vi "Get CAN Task Events.vi"(11 "CANopen Master in":refnum<class "CANopen Master.lvclass">) -> (2 "CAN Task Events":T1, 3 "CANopen Master out":refnum<class "CANopen Master.lvclass">)   [LabVIEW 2024, in "CANopen Master.lvlib" / "CANopen Master.lvclass"]
uses:
  CANopen Master.lvclass
  CANopen Master.lvclass/CANopen Master.ctl
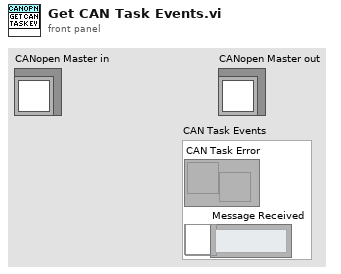
[diagram p1: front panel]
types:
  T1 = cluster{"CAN Task Error":refnum<user-event>, "Message Received":refnum<user-event>}
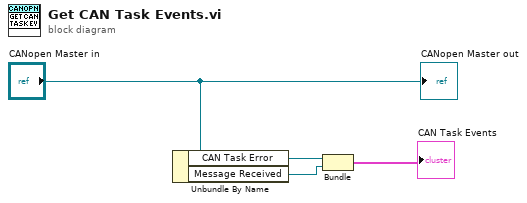
[diagram p0: block diagram]
diagram:
  n1 = Unbundle By Name("CANopen Master in") -> ("CAN Task Error"=w3:refnum<user-event>, "Message Received"=w2:refnum<user-event>)
  n2 = Bundle("CAN Task Error"=w3, "Message Received"=w2) -> (→"CAN Task Events":T1)  [unwired: 1 in]
  "CANopen Master out" <- "CANopen Master in"
